vi "optionsAcq_spectrumSmoothing.vi"(0 "reference":refnum<class "OSA.lvclass">, 2 "smoothing":T1, 4 "readWrite":enum16{"read", "write"}(ring), 5 "error in (no error)":errorcluster, 6 "width":u16, 7 "ignore range violation (false)":bool, 8 "nrOfPasses":u16) -> (10 "nrOfPasses out":u16, 12 "width out":u16, 14 "duplicate reference":refnum<class "OSA.lvclass">, 15 "status":string, 16 "smoothing out":T1, 19 "error out":errorcluster)   [LabVIEW 2010, in "OSA.lvclass"]
uses:
  OSA.lvclass
  FTSLib.dll
  typeDef/smoothing.ctl
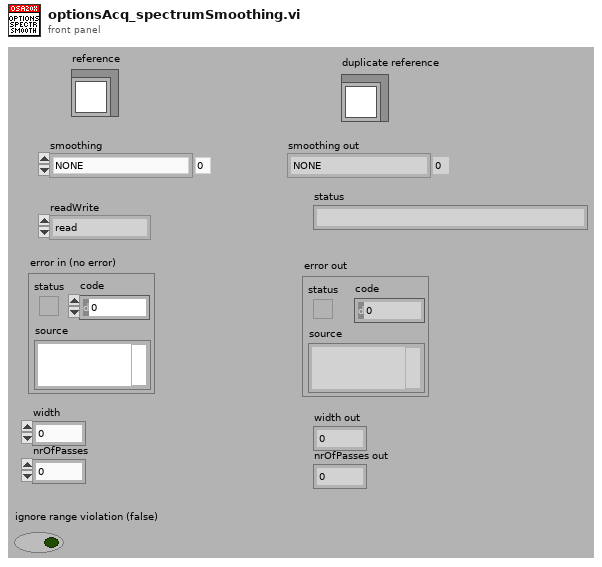
[diagram p1: front panel]
types:
  T1 = typedef "OSA.lvclass/smoothing.ctl" = enum16{"NONE", "BINOMIAL", "SAVITSKY_GOLAY", "FOURIER", "MOVING_AVERAGE", "GAUSSIAN"}
  T2 = typedef "OSA.lvclass/ObjectAttributes.ctl" = cluster{"Stop":bool, "dataType":T3, "spectrometerIdx":u16, "buffer size interferogram":i32, "interferogram":cluster{"new":bool, "plot_x_ min":sgl, "plot_x_max":sgl, "plot_y_min":sgl, "plot_y_max":sgl, "Graph Intrfrgrm":T4, "timeStamp":u32, "signal (%)":dbl, "traces":cluster{"idx":u32, "broadBand":bool, "monoChromatic":bool, "peakToPeakSignal":dbl, "peakToPeakPos":dbl}[], "traces idx last":i32}, "spectrum":cluster{"new":bool, "plot_x_min":sgl, "plot_x_max":sgl, "plot_unit_x":T5, "plot_unit_y":T6, "plot_y_min":sgl, "plot_y_max":sgl, "Graph Spectrum":T4, "timeStamp":u32, "X_VAL_OPTIONS":enum16{"MIN_MAX", "ARRAY"}, "traces":cluster{"idx":u32}[], "traces idx last":i32}, "Thorlabs_OSA_64.lvclass:queue_action.ctlqueue ref":refnum<queue>, "action":T7, "plot zoom step":dbl, "buffer semaphore":T8, "acq stopped":bool, "dataType active":T3, "temperature (degr C)":sgl, "pressure (hPa)":sgl, "rel humidity (%)":sgl, "settings":cluster{"resolution":T9, "sensitivity":T10, "Average":bool, "average nr":u32, "apodisation":T11, "acq delay (ms)":u32, "airMesure":T12, "wmtr on":bool, "intfgrm_smooth_width":u16, "intfgrm_smooth_nrOfPasses":u16, "intfgrm_smooth":T1, "phaseCorrection":T13, "zeroFill":u8, "spectr_smooth":T1, "spectr_smooth_width":u16, "spectr_smooth_nrOfPasses":u16, "resolution (/cm)":sgl, "REF wavelength, (nm)":dbl, "gain_idx":u16, "gainAuto":bool, "gain_relative":dbl, "PD sensitivity mode":T14, "PD senseMode implemented":bool, "SensorTemperature implemented":bool, "SensorPressure implemented":bool, "SensorHumidity implemented":bool}, "peaks position":sgl[], "peaks width":sgl[], "peaks height":sgl[], "peaks max nr":u32, "peaks latest nr":i32, "peaks new":bool, "power":dbl, "power new":bool, "path":string, "wavelength (WNr)":dbl, "wavelength new":bool, "buffer size spectrum":i32, "status":string, "VI reference":refnum<vi>, "funcPointer":u64, "libraryPointer":u64, "singleAcquisition":bool, "coherenceLength (cm)":dbl, "coherenceLength new":bool, "spectrometer model":string, "spectrometer serial nr":string, "peaks thld left":sgl[], "peaks thld right":sgl[], "coherenceLength error (cm)":dbl, "ADC bits":u16, "peaks position centroid":sgl[], "peaks height centroid":sgl[], "OSA series":T15, "channel":u16, "channels_nr":i32, "channel stiched":u32}
  T3 = typedef "OSA.lvclass/acq_dataType.ctl" = enum16{"none", "interferogram", "spectrum"}
  T4 = typedef "OSA.lvclass/graph_intensity.ctl" = refnum<vi>
  T5 = typedef "OSA.lvclass/spectrum_x_unit.ctl" = enum16{"wavenr/cm", "THz", "eV", "nm_air", "nm_vac"}
  T6 = typedef "OSA.lvclass/y_unit.ctl" = enum16{"ADC counts", "dBm pwr absolute", "dBm pwr density", "mW pwr absolute", "mW pwr density"}
  T7 = typedef "OSA.lvclass/queue_action.ctl" = enum16{"none", "stop", "GUI_plotInterferogram", "GUI_plotSpectrum", "GUI_plotInterferogramRescale", "GUI_plotSpectrumRescale", "GUI_plotInterferogramReset", "GUI_plotSpectrumReset", "GUI_plotInterferogramAutoScaleY", "GUI_plotSpectrumAutoScaleY", "GUI_plotInterferogramZoomOut", "GUI_plotSpectrumZoomOut", "GUI_plotInterferogramPane", "GUI_plotSpectrumPane", "GUI_plotInterferogramZoomMouse", "GUI_plotSpectrumZoomMouse", "ENVIRONMENT temperature", "ENVIRONMENT pressure", "MODE_resolution set", "MODE_resolution get", "MODE_sensitivity set", "MODE_sensitivity get", "MODE_PDTemperature set", "MODE_PDTemperature get", "REBOOT/RESET firmware", "ACQASYNC_acquireSingleSpectrum", "ACQASYNC_continuous start", "ACQASYNC_continuous stop\n", "ACQASYNC_get last interferogram", "ACQASYNC_get last spectrum", "ACQASYNC_get last waveNr", "ACQOPT_interferogram smoothing set", "ACQOPT_interferogram smoothing get", "ACQOPT_spectrum smoothing set", "ACQOPT_spectrum smoothing get", "ACQOPT_apodisation type set", "ACQOPT_apodisation type get", "ACQOPT_phase correction type set", "ACQOPT_phase correction type get", "ACQOPT_acqIntervall_set", "ACQOPT_acqIntervall_get", "ACQOPT_average spectrum set", "ACQOPT_average spectrum get", "ACQOPT_rolling average set", "ACQOPT_rolling average get", "ACQOPT_zero fill factor set", "ACQOPT_zero fill factor get", "ACQOPT_cycle counting set", "ACQOPT_cycle counting get", "ACQOPT_air measure option set", "ACQOPT_air measure option get", "ACQOPT_gainLevel auto get", "ACQOPT_gainLevel auto set", "ACQOPT_gainLevel get", "ACQOPT_gainLevel set", "ACQOPT_getAll", "INSTRUMENT_PROPERTY_range_WaveNr_min", "INSTRUMENT_PROPERTY_range_WaveNr_max", "INSTRUMENT_PROPERTY_reference_wavelength_cm^-1", "INSTRUMENT_PROPERTY_samplesPerRefPeriod", "INSTRUMENT_PROPERTY_resolution_waveNrPercm", "INSTRUMENT_PROPERTY_availableGainLevels", "INSTRUMENT_PROPERTY_status", "CONVERT", "ANALYSE_POWER", "ANALYSE_PEAKS", "ANALYSE_WAVELENGTH", "ANALYSE_SPECTRUM", "ANALYSE_INTERFEROGRAM", "ANALYSE_COHERENCE_LENGTH", "MATH", "MATH_power", "MATH_peaks", "FILE", "miscellaneous"}
  T8 = typedef "Semaphore RefNum" = refnum<k1>
  T9 = typedef "OSA.lvclass/resolution.ctl" = enum16{"low", "high"}
  T10 = typedef "OSA.lvclass/sensitivityMode.ctl" = enum16{"low", "low medium", "high medium", "high"}
  T11 = typedef "OSA.lvclass/apodisation.ctl" = enum16{"NONE", "NORTON_BEER_WEAK", "NORTON_BEER_MEDIUM", "NORTON_BEER_STRONG", "TRIANGULAR", "COSINE", "HANN", "HAMMING", "BLACKMANHARRIS3", "BLACKMANHARRIS4", "GAUSSIAN"}
  T12 = typedef "OSA.lvclass/airMeasure.ctl" = enum16{"TEMPERATURE", "PRESSURE"}
  T13 = typedef "OSA.lvclass/phaseCorrection.ctl" = enum16{"NONE", "MERTZ", "FORMAN", "MERTZ_FILE", "FORMAN_FILE", "FUTURE COMP."}
  T14 = typedef "OSA.lvclass/PDTemperatureMode.ctl" = enum16{"cool: better sensitivity/noise floor", "warm: extended wl range"}
  T15 = typedef "OSA_series.ctl" = enum16{"OSA200", "OSA300", "UNKNOWN"}
  T16 = typedef "OSA20X.lvclass/ObjectAttributes.ctl" = cluster{"Stop":bool, "dataType":T17, "spectrometerIdx":u16, "buffer size interferogram":i32, "interferogram":cluster{"new":bool, "plot_x_ min":sgl, "plot_x_max":sgl, "plot_y_min":sgl, "plot_y_max":sgl, "Graph Intrfrgrm":T18, "timeStamp":u32, "signal (%)":dbl, "traces":cluster{"idx":u32, "broadBand":bool, "monoChromatic":bool, "peakToPeakSignal":dbl, "peakToPeakPos":dbl}[], "traces idx last":i32}, "spectrum":cluster{"new":bool, "plot_x_min":sgl, "plot_x_max":sgl, "plot_unit_x":T19, "plot_unit_y":T20, "plot_y_min":sgl, "plot_y_max":sgl, "Graph Spectrum":T18, "timeStamp":u32, "X_VAL_OPTIONS":enum16{"MIN_MAX", "ARRAY"}, "traces":cluster{"idx":u32}[], "traces idx last":i32}, "Thorlabs_OSA_64.lvclass:queue_action.ctlqueue ref":refnum<queue>, "action":T21, "plot zoom step":dbl, "buffer semaphore":T8, "acq stopped":bool, "dataType active":T17, "temperature (degr C)":sgl, "pressure (hPa)":sgl, "rel humidity (%)":sgl, "settings":cluster{"resolution":T22, "sensitivity":T23, "Average":bool, "average nr":u32, "apodisation":T24, "acq delay (ms)":u32, "airMesure":T25, "wmtr on":bool, "intfgrm_smooth_width":u16, "intfgrm_smooth_nrOfPasses":u16, "intfgrm_smooth":T26, "phaseCorrection":T27, "zeroFill":u8, "spectr_smooth":T26, "spectr_smooth_width":u16, "spectr_smooth_nrOfPasses":u16, "resolution (/cm)":sgl, "REF wavelength, (nm)":dbl, "gain_idx":u16, "gainAuto":bool, "gain_relative":dbl, "PD sensitivity mode":T28, "PD senseMode implemented":bool, "SensorTemperature implemented":bool, "SensorPressure implemented":bool, "SensorHumidity implemented":bool}, "peaks position":sgl[], "peaks width":sgl[], "peaks height":sgl[], "peaks max nr":u32, "peaks latest nr":i32, "peaks new":bool, "power":dbl, "power new":bool, "path":string, "wavelength (WNr)":dbl, "wavelength new":bool, "buffer size spectrum":i32, "status":string, "VI reference":refnum<vi>, "funcPointer":u64, "libraryPointer":u64, "singleAcquisition":bool, "coherenceLength (cm)":dbl, "coherenceLength new":bool, "spectrometer model":string, "spectrometer serial nr":string, "peaks thld left":sgl[], "peaks thld right":sgl[], "coherenceLength error (cm)":dbl, "ADC bits":u16, "peaks position centroid":sgl[], "peaks height centroid":sgl[], "OSA series":T15, "channel":u16, "channels_nr":i32, "channel stiched":u32}
  T17 = typedef "OSA20X.lvclass/acq_dataType.ctl" = enum16{"none", "interferogram", "spectrum"}
  T18 = typedef "OSA20X.lvclass/graph_intensity.ctl" = refnum<vi>
  T19 = typedef "OSA20X.lvclass/spectrum_x_unit.ctl" = enum16{"wavenr/cm", "THz", "eV", "nm_air", "nm_vac"}
  T20 = typedef "OSA20X.lvclass/y_unit.ctl" = enum16{"ADC counts", "dBm pwr absolute", "dBm pwr density", "mW pwr absolute", "mW pwr density"}
  T21 = typedef "OSA20X.lvclass/queue_action.ctl" = enum16{"none", "stop", "GUI_plotInterferogram", "GUI_plotSpectrum", "GUI_plotInterferogramRescale", "GUI_plotSpectrumRescale", "GUI_plotInterferogramReset", "GUI_plotSpectrumReset", "GUI_plotInterferogramAutoScaleY", "GUI_plotSpectrumAutoScaleY", "GUI_plotInterferogramZoomOut", "GUI_plotSpectrumZoomOut", "GUI_plotInterferogramPane", "GUI_plotSpectrumPane", "GUI_plotInterferogramZoomMouse", "GUI_plotSpectrumZoomMouse", "ENVIRONMENT temperature", "ENVIRONMENT pressure", "MODE_resolution set", "MODE_resolution get", "MODE_sensitivity set", "MODE_sensitivity get", "MODE_PDTemperature set", "MODE_PDTemperature get", "REBOOT/RESET firmware", "ACQASYNC_acquireSingleSpectrum", "ACQASYNC_continuous start", "ACQASYNC_continuous stop\n", "ACQASYNC_get last interferogram", "ACQASYNC_get last spectrum", "ACQASYNC_get last waveNr", "ACQOPT_interferogram smoothing set", "ACQOPT_interferogram smoothing get", "ACQOPT_spectrum smoothing set", "ACQOPT_spectrum smoothing get", "ACQOPT_apodisation type set", "ACQOPT_apodisation type get", "ACQOPT_phase correction type set", "ACQOPT_phase correction type get", "ACQOPT_acqIntervall_set", "ACQOPT_acqIntervall_get", "ACQOPT_average spectrum set", "ACQOPT_average spectrum get", "ACQOPT_rolling average set", "ACQOPT_rolling average get", "ACQOPT_zero fill factor set", "ACQOPT_zero fill factor get", "ACQOPT_cycle counting set", "ACQOPT_cycle counting get", "ACQOPT_air measure option set", "ACQOPT_air measure option get", "ACQOPT_gainLevel auto get", "ACQOPT_gainLevel auto set", "ACQOPT_gainLevel get", "ACQOPT_gainLevel set", "ACQOPT_getAll", "INSTRUMENT_PROPERTY_range_WaveNr_min", "INSTRUMENT_PROPERTY_range_WaveNr_max", "INSTRUMENT_PROPERTY_reference_wavelength_cm^-1", "INSTRUMENT_PROPERTY_samplesPerRefPeriod", "INSTRUMENT_PROPERTY_resolution_waveNrPercm", "INSTRUMENT_PROPERTY_availableGainLevels", "INSTRUMENT_PROPERTY_status", "CONVERT", "ANALYSE_POWER", "ANALYSE_PEAKS", "ANALYSE_WAVELENGTH", "ANALYSE_SPECTRUM", "ANALYSE_INTERFEROGRAM", "ANALYSE_COHERENCE_LENGTH", "MATH", "MATH_power", "MATH_peaks", "FILE", "miscellaneous"}
  T22 = typedef "OSA20X.lvclass/resolution.ctl" = enum16{"low", "high"}
  T23 = typedef "OSA20X.lvclass/sensitivityMode.ctl" = enum16{"low", "low medium", "high medium", "high"}
  T24 = typedef "OSA20X.lvclass/apodisation.ctl" = enum16{"NONE", "NORTON_BEER_WEAK", "NORTON_BEER_MEDIUM", "NORTON_BEER_STRONG", "TRIANGULAR", "COSINE", "HANN", "HAMMING", "BLACKMANHARRIS3", "BLACKMANHARRIS4", "GAUSSIAN"}
  T25 = typedef "OSA20X.lvclass/airMeasure.ctl" = enum16{"TEMPERATURE", "PRESSURE"}
  T26 = typedef "OSA20X.lvclass/smoothing.ctl" = enum16{"NONE", "BINOMIAL", "SAVITSKY_GOLAY", "FOURIER", "MOVING_AVERAGE", "GAUSSIAN"}
  T27 = typedef "OSA20X.lvclass/phaseCorrection.ctl" = enum16{"NONE", "MERTZ", "FORMAN", "MERTZ_FILE", "FORMAN_FILE", "FUTURE COMP."}
  T28 = typedef "OSA20X.lvclass/PDTemperatureMode.ctl" = enum16{"cool: better sensitivity/noise floor", "warm: extended wl range"}
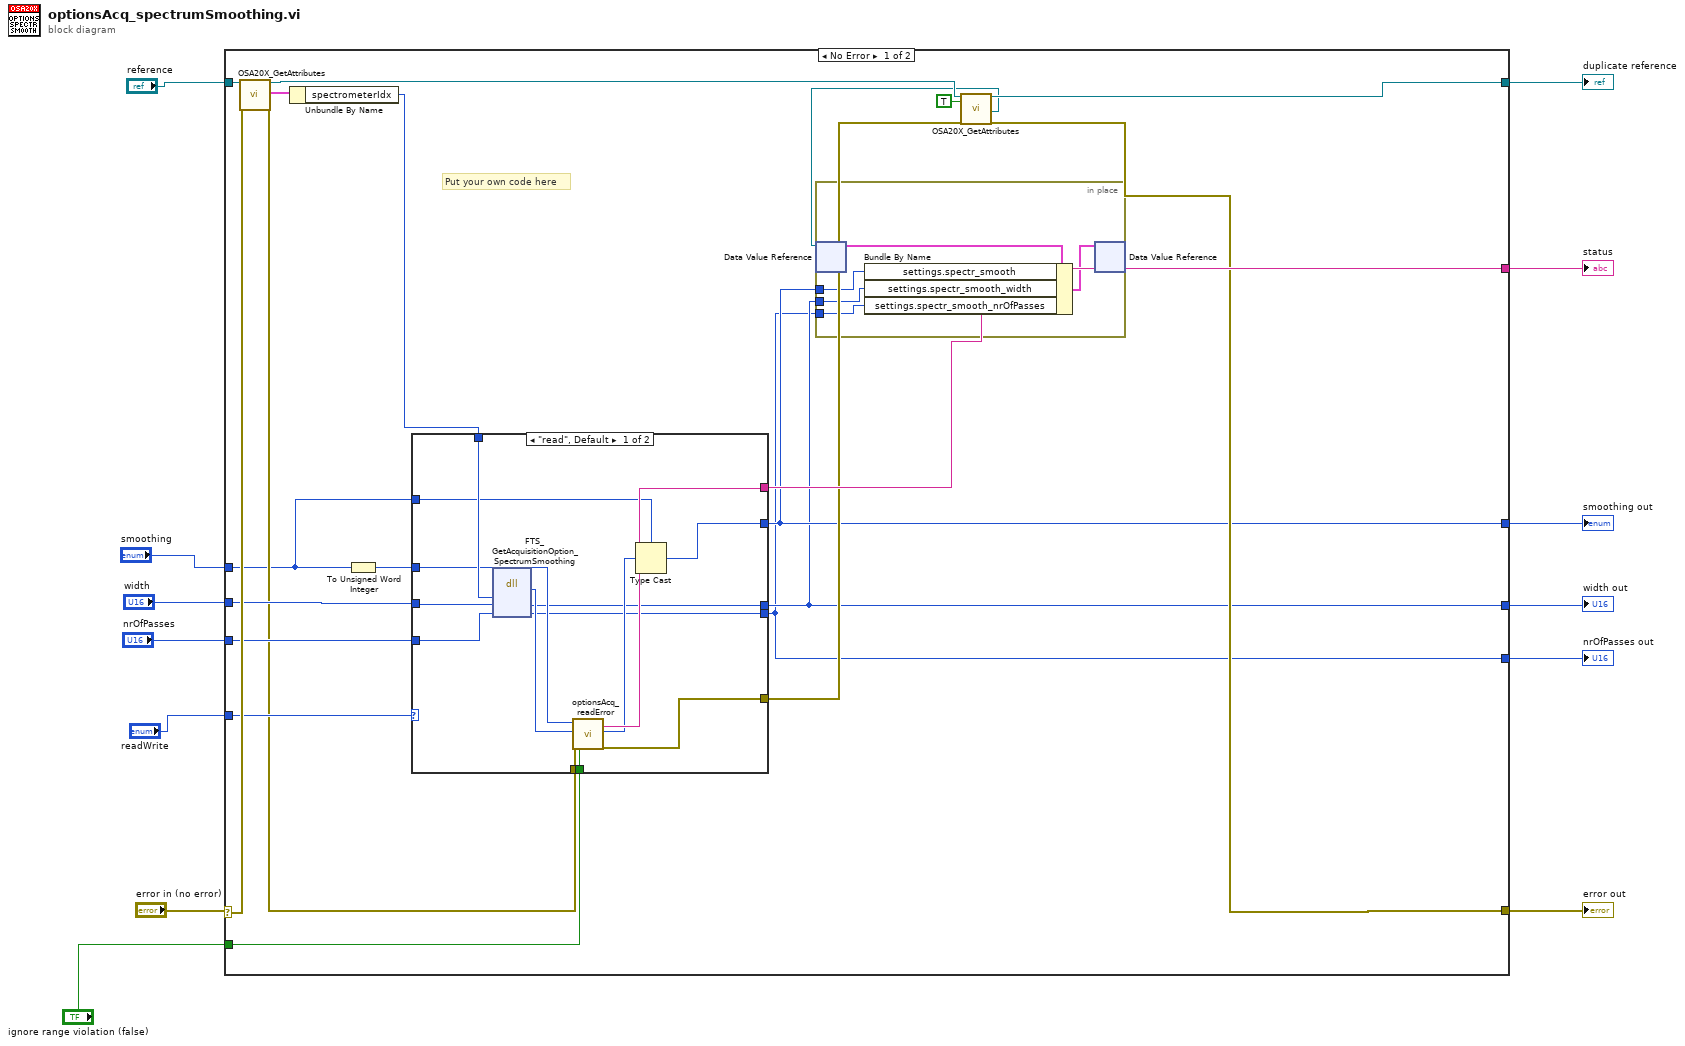
[diagram p0: block diagram]
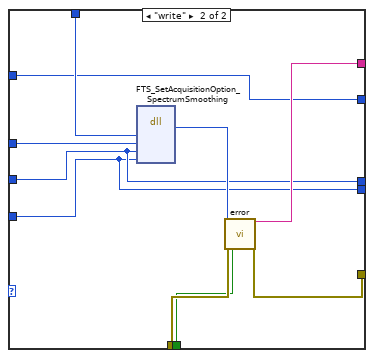
[diagram p2: hidden frame]
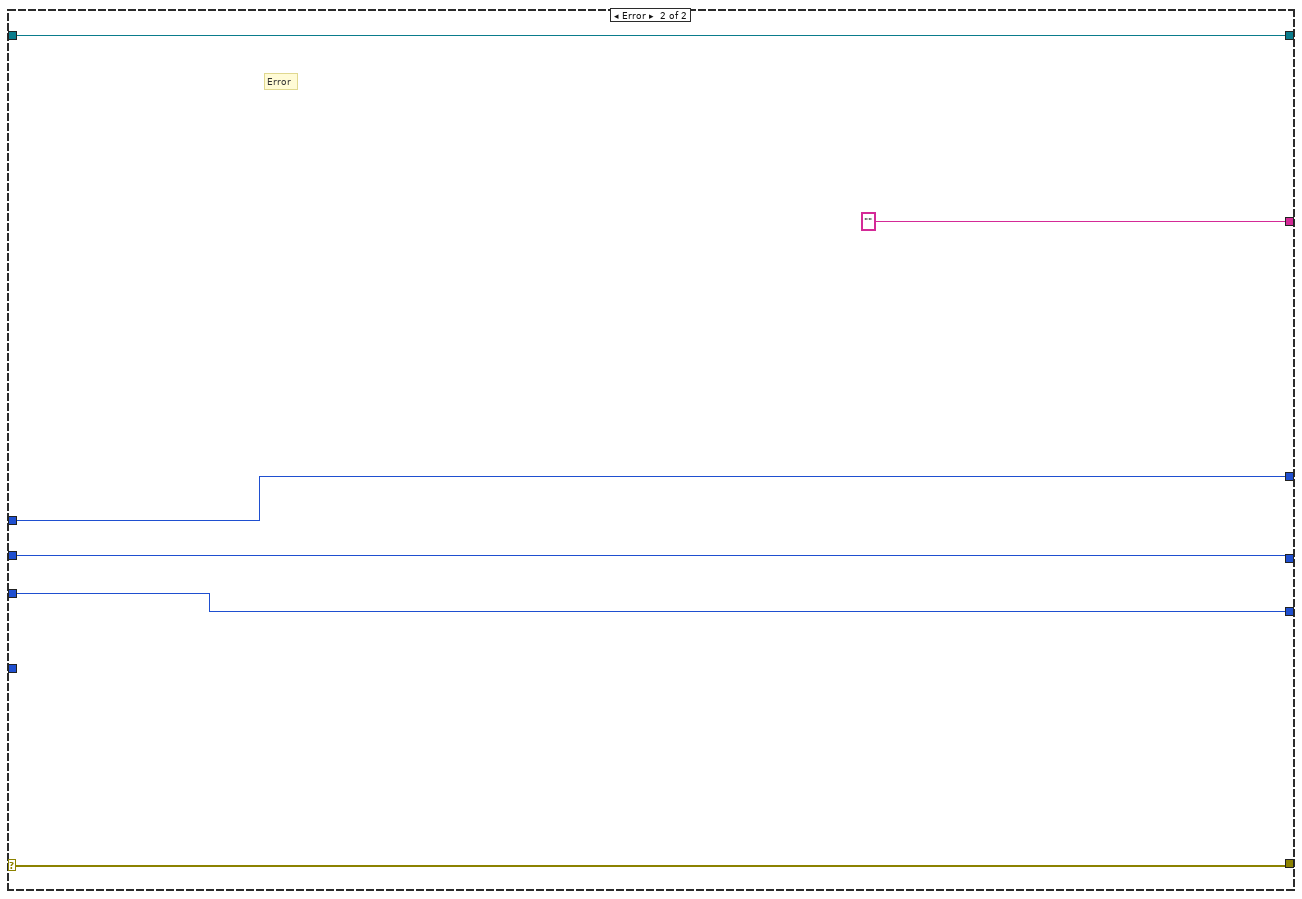
[diagram p3: hidden frame]
diagram:
  n1 = case shown="No Error" "error in (no error)" {
    selector: "error in (no error)" -> [w33 w68]
    tunnel: [w20 w68] -> w13
    tunnel: "reference" -> [w34 w69]
    tunnel: [w23 w69] -> w10
    tunnel: "readWrite" -> [w31 _]
    tunnel: "smoothing" -> [w24 w64]
    tunnel: "width" -> [w29 w66]
    tunnel: "nrOfPasses" -> [w28 w65]
    tunnel: [w26 "" ("status")] -> w5
    tunnel: [w15 w66] -> w4
    tunnel: [w14 w65] -> w3
    tunnel: "ignore range violation (false)" -> [w25 _]
    tunnel: [w16 w64] -> w1
    frame No Error {
      # "Put your own code here"
      n2 = call "OSA20X_GetAttributes.vi"("reference in"=w34, "error in (no error)"=w33) -> ("reference out"=w22:refnum<class "OSA.lvclass">, "Data"=w18:T2, "error out"=w27:errorcluster)  [unwired: 14 in, 1 out]
      n3 = Unbundle By Name(w18) -> ("spectrometerIdx"=w32:u16)
      n4 = To Unsigned Word Integer(number=w24) -> (unsigned 16bit integer=w30:u16)
      n5 = case shown="\"read\", Default" w31 {
        tunnel: w32 -> [w53 w63]
        tunnel: w30 -> [w47 w62]
        tunnel: w29 -> [w52 w55]
        tunnel: w28 -> [w51 w54]
        tunnel: [w42 w55] -> w15
        tunnel: [w41 w54] -> w14
        tunnel: w27 -> [w50 w60]
        tunnel: [w40 w59] -> w21
        tunnel: [w46 w58] -> w26
        tunnel: w25 -> [w49 w57]
        tunnel: [w43 w56] -> w16
        tunnel: w24 -> [w44 w56]
        frame "read", Default {
          n6 = dll-call lib="FTSLib.dll" fn="FTS_GetAcquisitionOption_SpectrumSmoothing"("spectrIdx"=w53, "width"=w52, "nrOfPAsses"=w51) -> ("return type"=w48:i32, "width"=w42:u16, "nrOfPAsses"=w41:u16)  [unwired: 4 in, 2 out]
          n7 = call "optionsAcq_readError.vi"("option default"=w47, "option return"=w48, "error in (no error)"=w50, "error ignore"=w49) -> ("status"=w46:string, "option"=w45:u16, "error out"=w40:errorcluster)  [unwired: 13 in]
          n8 = Type Cast(type=w44, x=w45) -> (*(type *) &x=w43:T1)
        }
        frame "write" {
          n9 = dll-call lib="FTSLib.dll" fn="FTS_SetAcquisitionOption_SpectrumSmoothing"("spectrIdx"=w63, "smoothingType"=w62, "width"=w55, "nrOfPasses"=w54) -> ("return type"=w61:i32)  [unwired: 7 in, 2 out]
          n10 = call "error.vi"("result code"=w61, "error in (no error)"=w60, "ignore range violation"=w57) -> ("status"=w58:string, "error out"=w59:errorcluster)  [unwired: 14 in, 1 out]
        }
      }
      n11 = call "OSA20X_GetAttributes.vi"("reference in"=w22, "OnlyGetDvrReference(False)"=TRUE, "error in (no error)"=w21) -> ("reference out"=w23:refnum<class "OSA.lvclass">, "DataRef"=w17:refnum<data-value>, "error out"=w20:errorcluster)  [unwired: 13 in, 1 out]
      n12 = in-place {
        in-place-border: w16 -> [w38]
        in-place-border: w15 -> [w37]
        in-place-border: w14 -> [w36]
        n13 = in-place-dvr #1(w17) -> (w39:T16)  [unwired: 1 out]
        n14 = Bundle By Name(cluster=w39, "settings.spectr_smooth"=w38, "settings.spectr_smooth_width"=w37, "settings.spectr_smooth_nrOfPasses"=w36) -> (w35:T16)
        n15 = in-place-dvr #1(w35) -> ()  [unwired: 2 out]
      }
    }
    frame Error {
      # "Error"
    }
  }
  "error out" <- w13
  "duplicate reference" <- w10
  "status" <- w5
  "nrOfPasses out" <- w3
  "width out" <- w4
  "smoothing out" <- w1
